vi "Gray_Binary.vi"() -> ()   [LabVIEW 2024]
panel:
  out "b0":bool
  in  "g0":bool
  out "b1":bool
  in  "g1":bool
  out "b3":bool
  in  "g2":bool
  out "b2":bool
  in  "g3":bool
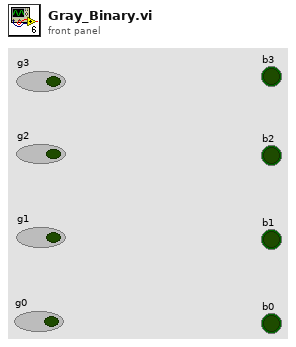
[diagram p1: front panel]
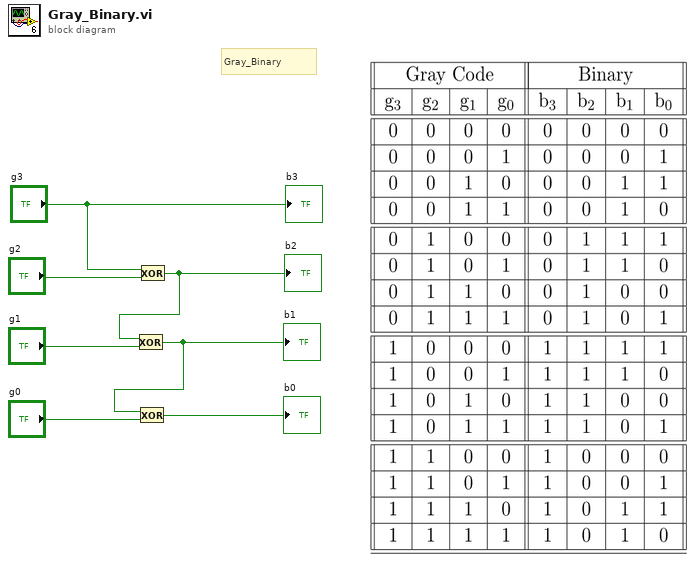
[diagram p0: block diagram]
diagram:
  # "Gray_Binary"
  n1 = Exclusive Or(1:"g2", 2:"g3") -> (0:w2:bool)
  "b2" <- w2
  n2 = Exclusive Or(1:"g1", 2:w2) -> (0:w1:bool)
  "b1" <- w1
  n3 = Exclusive Or(1:"g0", 2:w1) -> (0:→"b0":bool)
  "b3" <- "g3"
